vi "Create Data File.vi"(6 "File Type":enum16{"text (.txt)", "Excel Workbook (.xlsx)"}(ring), 7 "base path":path=path "C:/LFO/Electrical Test Results", 8 "error in (no error)":errorcluster, 9 "Description":string="Raw", 10 "Serial Number":string="2163", 11 "Part Number":string="2163") -> (0 "error out (no error)":errorcluster, 2 "File Path Out":path)   [LabVIEW 2018]
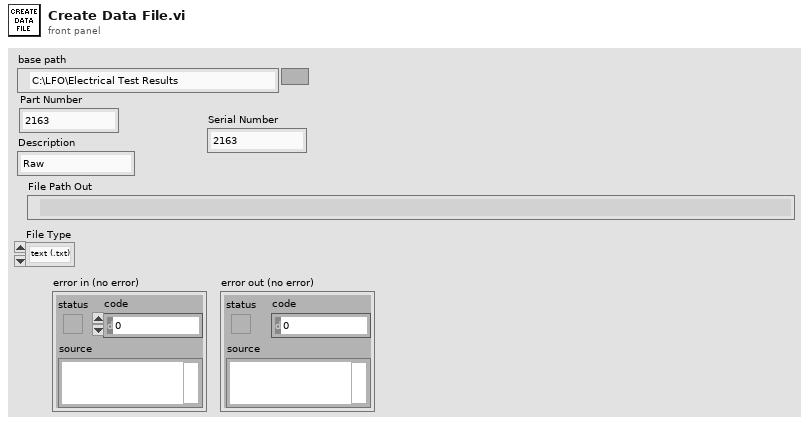
[diagram p1: front panel]
types:
  T1 = enum16{"open", "replace", "create", "open or create", "replace or create", "replace or create with confirmation"}
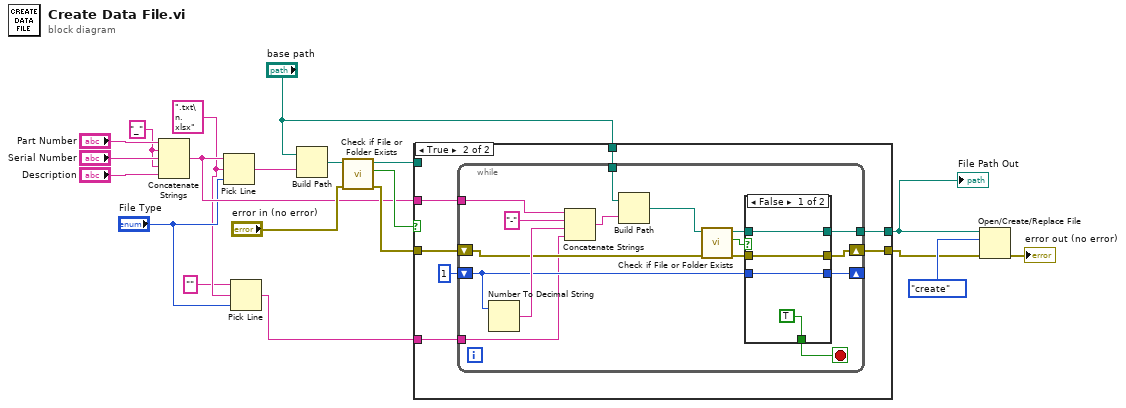
[diagram p0: block diagram]
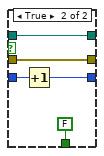
[diagram p3: hidden frame]
diagram:
  w3 = ".txt\n.xlsx" ("multi-line string")
  w18 = "_" ("string")
  n1 = Concatenate Strings("Part Number", w18, "Serial Number", w18, "Description") -> (w6:string)
  n2 = Pick Line(string ("")=w6, multi-line string=w3, line index="File Type") -> (output string=w5:string)
  n3 = Pick Line(string ("")="", multi-line string=w3, line index="File Type") -> (output string=w1:string)
  n4 = Build Path(base path="base path", name or relative path=w5) -> (appended path=w12:path)
  n5 = call <vilib>:"Check if File or Folder Exists.vi"("error in (no error)"="error in (no error)", "path"=w12) -> ("error out"=w9:errorcluster, "file or folder exists?"=w15:bool, "dup path"=w16:path)  [unwired: 7 in]
  n6 = case shown="True" w15 {
    tunnel: [w22 w29] -> w14
    tunnel: w16 -> [w22 _]
    tunnel: w6 -> [_ w27]
    tunnel: "base path" -> [_ w26]
    tunnel: w9 -> [w21 w25]
    tunnel: [w21 w24] -> w8
    tunnel: w1 -> [_ w23]
    frame False {
    }
    frame True {
      n7 = while {
        tunnel: [w39] -> w29
        shift-right: [w37] -> _
        shift-left: i64 1 ("Sample #") -> [w38]
        tunnel: w27 -> [w35]
        tunnel: w26 -> [w34]
        shift-right: [w32] -> w24
        shift-left: w25 -> [w33]
        tunnel: w23 -> [w30]
        stop <- w36 stop-if-true
        n8 = Number To Decimal String(number=w38) -> (decimal integer string=w43:string)  [unwired: 1 in]
        n9 = Concatenate Strings(w35, "-" ("string"), w43, w30) -> (w45:string)
        n10 = Build Path(base path=w34, name or relative path=w45) -> (appended path=w40:path)
        n11 = call <vilib>:"Check if File or Folder Exists.vi"("error in (no error)"=w33, "path"=w40) -> ("error out"=w31:errorcluster, "file or folder exists?"=w42:bool, "dup path"=w41:path)  [unwired: 7 in]
        n12 = case shown="False" w42 {
          tunnel: [w49 w54] -> w39
          tunnel: w41 -> [w49 w54]
          tunnel: w38 -> [w48 w53]
          tunnel: [w48 w52] -> w37
          tunnel: [TRUE FALSE] -> w36
          tunnel: [w46 w50] -> w32
          tunnel: w31 -> [w46 w50]
          frame False {
          }
          frame True {
            n13 = Increment(x=w53) -> (x+1=w52:i64)
          }
        }
      }
    }
  }
  "File Path Out" <- w14
  n14 = Open/Create/Replace File(file path (use dialog)=w14, error in=w8, operation (0:open)=T1."create") -> (error out=→"error out (no error)":errorcluster)  [unwired: 3 in, 2 out]
